vi "FR Measure.vi"(11 "FFmeter settings":T1={"AC Source"={"AC Source type"=enum."Fluke 5XXX calibrator", "VISA"="", "Ref. clock (Hz)"=0.0, "status ref"=refnum}, "TWM pipe"="\\\\.\\pipe\\TWM:server", "Measurement status ref"=refnum, "TWM Status ref"=refnum, "Abort ref"=refnum, "DC meter"={"DC meter type"=enum."H/A/K 3458", "DC meter VISA"="", "NPLC"=10, "status ref"=refnum}, "Measurement properties"={"Measurement frequencies (Hz)"=[1000.0], "Sampling frequency (Hz)"=500000.0, "Signal amplitude (V)"=4.5, "AC-DC settle time (s)"=20.0, "Record length (multiples of period)"=[1000.0, 10000.0, 1000.0], "Measurement template file"=path "", "Row of START keyword"=1, "Row of STOP keyword"=0, "Calculate RMS from samples"=FALSE, "AC-DC warm up time (s)"=300.0, "Measurement template line"=[], "DC meter readings No."=10, "Algorithm"="TWM-WFFT"}, "Skip waiting ref"=refnum, "Octave paths"={"GNU Octave path"=path "C:/Program Files/GNU Octave/Octave-6.2.0/mingw64/bin", "TWM+QWTB path"=path "C:/Users/labina/Desktop/TWM-1.8.7.0-full/octprog", "lvlib path"=path "D:/martin/WAC/WACsw - github/control_software/Filter function meter/external libraries/GOLPI 0.7.3.1 source distribution LV 20.0 32 bit/lv_proc.dll"}, "Template definition"={"Keywords column"=0, "Sig. freq. column"=1, "Rec. len. column"=2, "Meas. points. row min to read"=9, "Meas. points. row max to read"=1509, "Properties column"=4, "Properties row start"=1, "Properties row end"=5, "Keyword START regexp"="", "Keyword STOP regexp"="", "HW data column"=7, "HW data row start"=1, "HW data row end"=3, "TIme and date column start"=3, "Digitizer value column start "=4, "DC mean column start "=6, "DC readings column start"=10}} {"Measurement properties"."Record length (multiples of period)" format="%#_3p"; "Measurement properties"."Sampling frequency (Hz)" format="%#_3p"; "Measurement properties"."Measurement frequencies (Hz)" format="%#_3p"}) -> (0 "error out":errorcluster, 3 "FFmeter settings out":T1={"AC Source"={"AC Source type"=enum."Fluke 5XXX calibrator", "VISA"="", "Ref. clock (Hz)"=0.0, "status ref"=refnum}, "TWM pipe"="\\\\.\\pipe\\TWM:server", "Measurement status ref"=refnum, "TWM Status ref"=refnum, "Abort ref"=refnum, "DC meter"={"DC meter type"=enum."H/A/K 3458", "DC meter VISA"="", "NPLC"=10, "status ref"=refnum}, "Measurement properties"={"Measurement frequencies (Hz)"=[1000.0], "Sampling frequency (Hz)"=500000.0, "Signal amplitude (V)"=4.5, "AC-DC settle time (s)"=20.0, "Record length (multiples of period)"=[1000.0, 10000.0, 1000.0], "Measurement template file"=path "", "Row of START keyword"=1, "Row of STOP keyword"=0, "Calculate RMS from samples"=FALSE, "AC-DC warm up time (s)"=300.0, "Measurement template line"=[], "DC meter readings No."=10, "Algorithm"="TWM-WFFT"}, "Skip waiting ref"=refnum, "Octave paths"={"GNU Octave path"=path "C:/Program Files/GNU Octave/Octave-6.2.0/mingw64/bin", "TWM+QWTB path"=path "C:/Users/labina/Desktop/TWM-1.8.7.0-full/octprog", "lvlib path"=path "D:/martin/WAC/WACsw - github/control_software/Filter function meter/external libraries/GOLPI 0.7.3.1 source distribution LV 20.0 32 bit/lv_proc.dll"}, "Template definition"={"Keywords column"=0, "Sig. freq. column"=1, "Rec. len. column"=2, "Meas. points. row min to read"=9, "Meas. points. row max to read"=1509, "Properties column"=4, "Properties row start"=1, "Properties row end"=5, "Keyword START regexp"="", "Keyword STOP regexp"="", "HW data column"=7, "HW data row start"=1, "HW data row end"=3, "TIme and date column start"=3, "Digitizer value column start "=4, "DC mean column start "=6, "DC readings column start"=10}} {"Measurement properties"."Record length (multiples of period)" format="%#_3p"; "Measurement properties"."Sampling frequency (Hz)" format="%#_3p"; "Measurement properties"."Measurement frequencies (Hz)" format="%#_3p"})   [LabVIEW 2020]
uses:
  FR GUI/Type definitions/FFmeter settings.ctl
  General AC source/Type definitions/AC Source.ctl
  General AC source/Type definitions/AC Source type.ctl
  General DC meter/Type definitions/DC meter.ctl
  General DC meter/Type definitions/DC meter type.ctl
  Type definitions/FR Measuement properties.ctl
  FR Utilities/Type definitions/FR Template definition.ctl
  <vilib>/Utility/error.llb/DialogType.ctl
  external libraries/TWM-1.8.7.0-client/TWM Client Quantity Record.ctl
  <vilib>/Utility/NIReport.llb/NI_report.lvclass
  external libraries/varilib/varilib.lvlib
  external libraries/TWM-1.8.7.0-client/TWM Client.lvlib
panel:
  out "DC readings of AC-AC sequence":dbl[][](array[numeric])
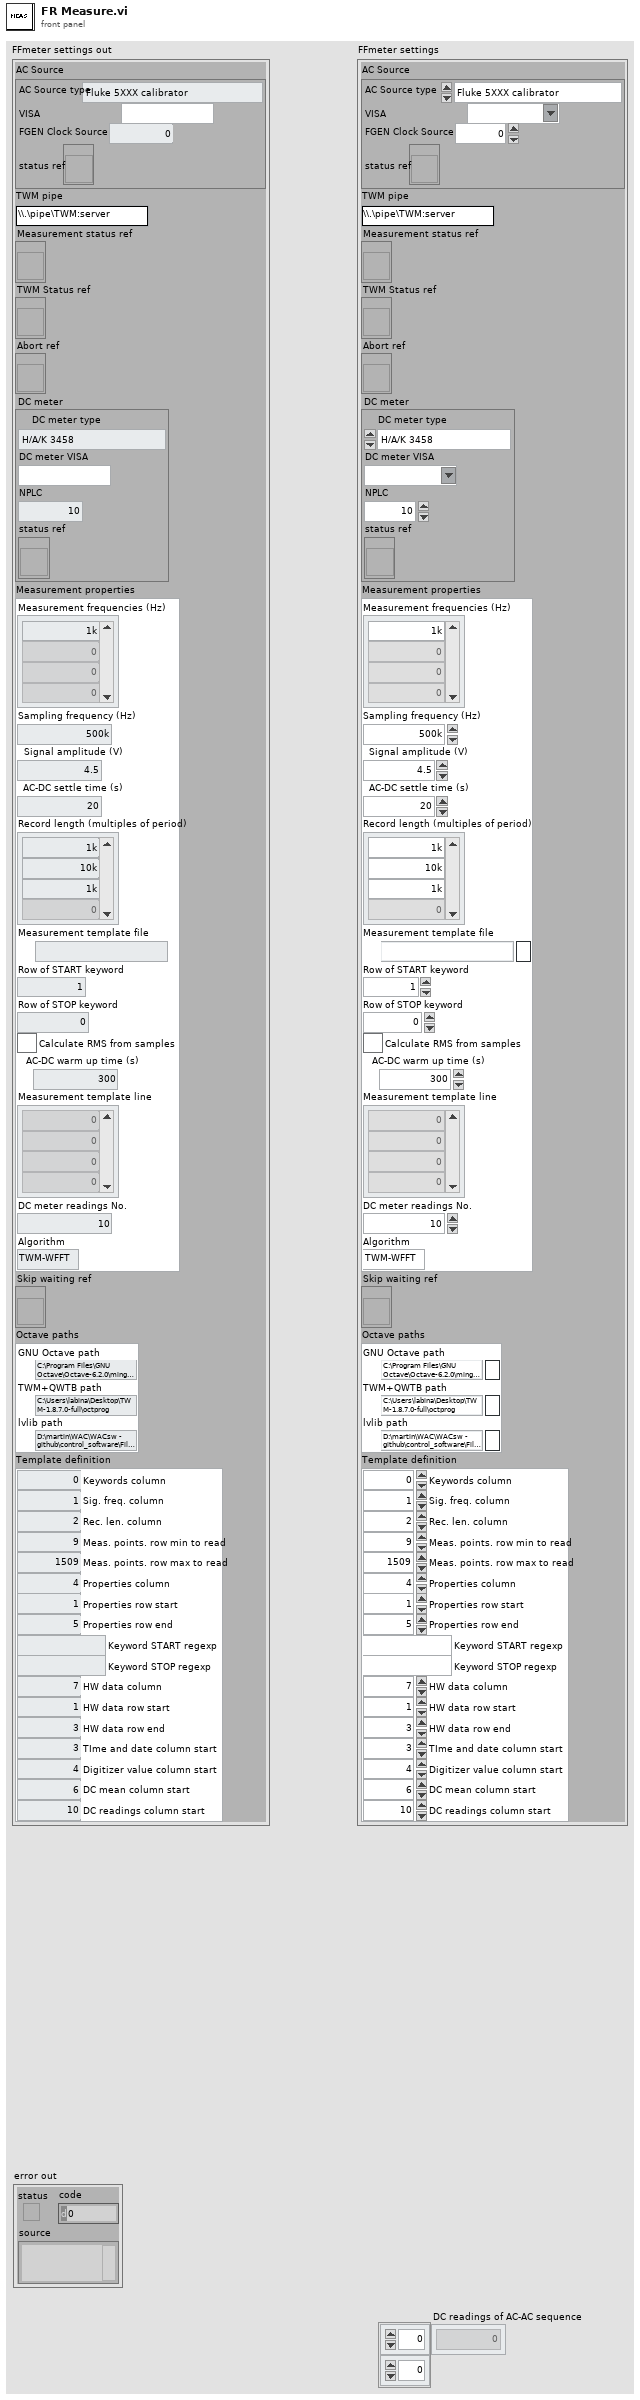
[diagram p1: front panel]
types:
  T1 = typedef "FFmeter settings.ctl" = cluster{"AC Source":T2, "TWM pipe":string, "Measurement status ref":refnum<vi>, "TWM Status ref":refnum<vi>, "Abort ref":refnum<vi>, "DC meter":T4, "Measurement properties":T6, "Skip waiting ref":refnum<vi>, "Octave paths":cluster{"GNU Octave path":path, "TWM+QWTB path":path, "lvlib path":path}, "Template definition":T7}
  T2 = typedef "AC Source.ctl" = cluster{"AC Source type":T3, "VISA":refnum<visa-resource-name>, "Ref. clock (Hz)":dbl, "status ref":refnum<vi>}
  T3 = typedef "AC Source type.ctl" = enum16{"Fluke 5XXX calibrator", "Tektronix AFG3000 series", "dummy"}
  T4 = typedef "DC meter.ctl" = cluster{"DC meter type":T5, "DC meter VISA":refnum<visa-resource-name>, "NPLC":i32, "status ref":refnum<vi>}
  T5 = typedef "DC meter type.ctl" = enum16{"H/A/K 3458", "FLuke 8508A", "dummy"}
  T6 = typedef "FR Measuement properties.ctl" = cluster{"Measurement frequencies (Hz)":dbl[], "Sampling frequency (Hz)":dbl, "Signal amplitude (V)":dbl, "AC-DC settle time (s)":dbl, "Record length (multiples of period)":dbl[], "Measurement template file":path, "Row of START keyword":i32, "Row of STOP keyword":i32, "Calculate RMS from samples":bool, "AC-DC warm up time (s)":dbl, "Measurement template line":i32[], "DC meter readings No.":i32, "Algorithm":string}
  T7 = typedef "FR Template definition.ctl" = cluster{"Keywords column":i32, "Sig. freq. column":i32, "Rec. len. column":i32, "Meas. points. row min to read":i32, "Meas. points. row max to read":i32, "Properties column":i32, "Properties row start":i32, "Properties row end":i32, "Keyword START regexp":string, "Keyword STOP regexp":string, "HW data column":i32, "HW data row start":i32, "HW data row end":i32, "TIme and date column start":i32, "Digitizer value column start ":i32, "DC mean column start ":i32, "DC readings column start":i32}
  T8 = typedef "DialogType.ctl" = u16
  T9 = typedef "TWM Client.lvlib/TWM Client Quantity Record.ctl" = cluster{"val":dbl[], "unc":dbl[], "name":string, "is valid?":bool, "has unc?":bool, "numel":i32, "ua":dbl[], "is phase?":bool, "is amplitude?":bool, "description":string, "phase tag":string, "num format":string, "is string?":bool, "string value":string}
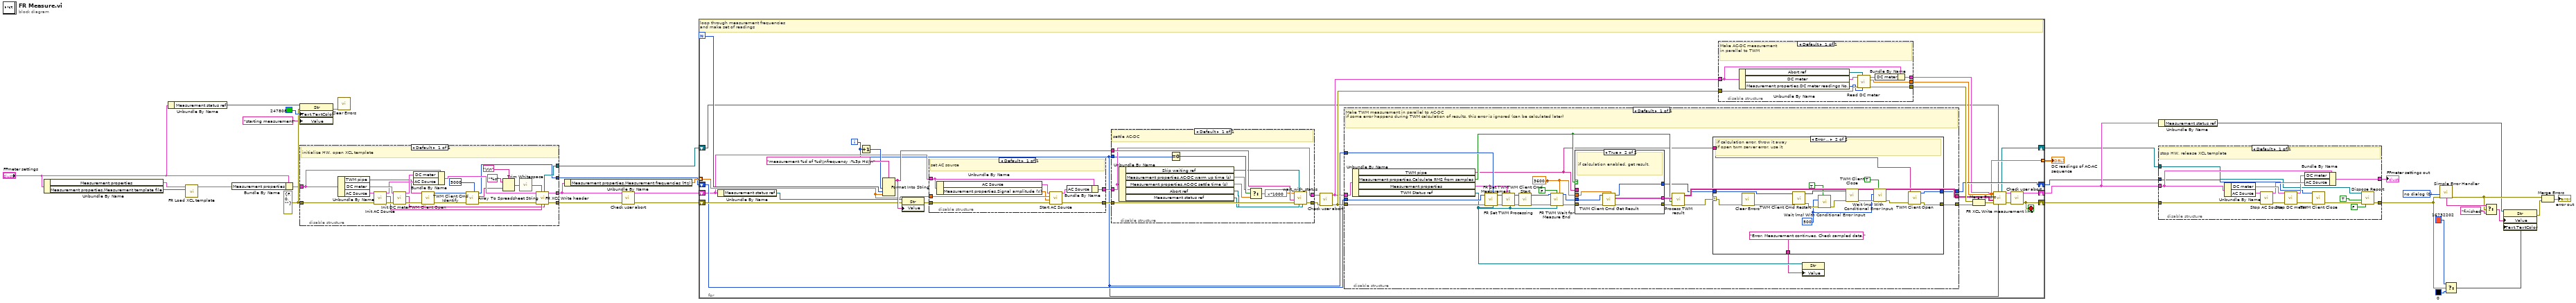
[diagram p0: block diagram]
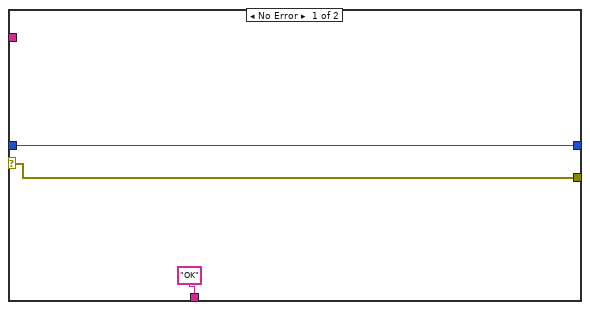
[diagram p2: hidden frame]
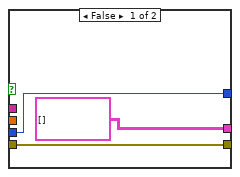
[diagram p3: hidden frame]
diagram:
  w30 = T8 0 items=["no dialog", "OK message", "continue or stop message", "OK message + warnings", "continue/stop + warnings"] ("type of dialog (OK msg:1)")
  w10 = errorcluster {"status"=FALSE, "code"=0, "source"=""} ("error out")
  n1 = Unbundle By Name("FFmeter settings") -> ("Measurement properties"=w8:T6, "Measurement properties.Measurement template file"=w4:path)
  n2 = Unbundle By Name("FFmeter settings") -> ("Measurement status ref"=w22:refnum<vi>)
  n3 = call "FR Load XCL template.vi"("Measurement template file"=w4, "Measurement properties"=w8) -> ("Measurement properties out"=w7:T6)  [unwired: 9 in]
  n4 = Bundle By Name(cluster="FFmeter settings", "Measurement properties"=w7) -> (w5:T1)
  n5 = property class="Str"(reference=w22, error in=w10, "Text.TextColor"=u32 247808 ("Text.Text Colors:Text Color"), "Value"="starting measurement") -> (error out=w21:errorcluster)  [unwired: 1 out]
  n6 = disable-structure shown="Default" {
    disable-tunnel: w5 -> [w57]
    disable-tunnel: [w48] -> w1
    disable-tunnel: w10 -> [w54]
    disable-tunnel: [w51] -> w2
    disable-tunnel: [w39] -> w3
    disable-tunnel: [w49] -> w12
    frame Enabled {
      # "initialize HW, open XCL template"
      n7 = Unbundle By Name(w57) -> ("TWM pipe"=w52:string, "DC meter"=w58:T4, "AC Source"=w59:T2)
      n8 = call "Init AC Source.vi"("error in (no error)"=w54, "AC source"=w59) -> ("error out"=w60:errorcluster, "Init status"=w47:string, "AC source out"=w55:T2)  [unwired: 7 in]
      n9 = call "Init DC meter.vi"("error in (no error)"=w60, "DC meter"=w58) -> ("error out"=w53:errorcluster, "Init status"=w46:string, "DC meter out"=w56:T4)  [unwired: 7 in]
      n10 = Bundle By Name(cluster=w57, "DC meter"=w56, "AC Source"=w55) -> (w50:T1)
      n11 = call "TWM Client Open.vi"("error in"=w53, "pipe name"=w52) -> ("error out"=w41:errorcluster, "handle out"=w42:i32)  [unwired: 8 in]
      n12 = call "TWM Client Cmd Identify.vi"("timeout [ms]"=5000, "error in"=w41, "handle"=w42) -> ("error out"=w40:errorcluster, "channel idns"=w45:string[], "handle out"=w39:i32)  [unwired: 5 in, 1 out]
      n13 = Array To Spreadsheet String(delimiter (Tab)="\r\n", array=w45, 3:"%s" ("format string")) -> (spreadsheet string=w38:string)
      n14 = call <vilib>:"Trim Whitespace.vi"("string"=w38) -> ("trimmed string"=w37:string)  [unwired: 1 in]
      n15 = call "FR XCL Write header.vi"("DC meter idn"=w46, "AC source idn"=w47, "Digitizer idn"=w37, "error in (no error)"=w40, "FFmeter settings"=w50) -> ("error out"=w51:errorcluster, "FFmeter settings out"=w48:T1, "NI_report out"=w49:refnum<class "NI_report.lvclass">)  [unwired: 4 in]
    }
  }
  n16 = call <vilib>:"Clear Errors.vi"("error in (no error)"=w21) -> ()  [unwired: 5 in, 2 out]
  n17 = Unbundle By Name(w1) -> ("Measurement properties.Measurement frequencies (Hz)"=w35:dbl[])
  n18 = call "Check user abort.vi"("error in (no error)"=w2, "FFmeter settings"=w1) -> ("error out"=w20:errorcluster, "FFmeter settings out"=w19:T1)  [unwired: 8 in]
  n19 = for {
    N -> [w87]
    shift-right: [w74] -> w17
    shift-left: w20 -> [w79]
    shift-right: [w73] -> w15
    shift-left: w19 -> [w62]
    tunnel: w35 -> [w80] mode=indexing
    tunnel: [w70] -> w34 mode=indexing
    shift-right: [w66] -> w11
    shift-left: w12 -> [w65]
    shift-right: [w72] -> w13
    shift-left: w3 -> [w63]
    i -> [w61]
    stop <- w74 stop-if-true
    # "loop through measurement frequencies\nand make set of readings"
    n20 = Unbundle By Name(w62) -> ("Measurement status ref"=w84:refnum<vi>)
    n21 = Increment(x=w61) -> (x+1=w88:i32)
    n22 = Format Into String(format string="measurement %d of %d\\nfrequency :%3p Hz\\n", w88, w87, w80) -> (resulting string=w89:string)  [unwired: 2 in, 1 out]
    n23 = property class="Str"(reference=w84, error in=w79, "Value"=w89) -> (error out=w83:errorcluster)  [unwired: 1 out]
    n24 = disable-structure shown="Default" {
      disable-tunnel: w62 -> [w110]
      disable-tunnel: w83 -> [w109]
      disable-tunnel: [w108] -> w82
      disable-tunnel: [w111] -> w81
      disable-tunnel: w80 -> [w105]
      frame Enabled {
        # "set AC source"
        n25 = Unbundle By Name(w110) -> ("AC Source"=w106:T2, "Measurement properties.Signal amplitude (V)"=w104:dbl)
        n26 = call "Start AC Source.vi"("error in (no error)"=w109, "Signal amplitude (V)"=w104, "Signal frequency  (Hz)"=w105, "AC source"=w106) -> ("error out"=w108:errorcluster, "AC source out"=w107:T2)  [unwired: 5 in, 1 out]
        n27 = Bundle By Name(cluster=w110, "AC Source"=w107) -> (w111:T1)
      }
    }
    n28 = disable-structure shown="Default" {
      disable-tunnel: w89 -> [w103]
      disable-tunnel: [w97] -> w78
      disable-tunnel: [w101] -> w75
      disable-tunnel: w82 -> [w102]
      disable-tunnel: w81 -> [w101]
      disable-tunnel: w61 -> [w96]
      frame Enabled {
        # "settle AC-DC"
        n29 = Unbundle By Name(w101) -> ("Skip waiting ref"=w91:refnum<vi>, "Measurement properties.AC-DC warm up time (s)"=w94:dbl, "Measurement properties.AC-DC settle time (s)"=w93:dbl, "Abort ref"=w99:refnum<vi>, "Measurement status ref"=w98:refnum<vi>)
        n30 = Equal To 0?(x=w96) -> (x = 0?=w95:bool)
        n31 = Select(t=w94, s=w95, f=w93) -> (s? t:f=w92:dbl)
        n32 = expression code="x*1000"(w92) -> (w100:dbl)
        n33 = call "wait_with_status.vi"("stat ref"=w98, "stop ref"=w99, "second stop ref"=w91, "error in"=w102, "comment"=w103, "ms to wait"=w100) -> ("error out"=w97:errorcluster)  [unwired: 4 in, 1 out]
      }
    }
    n34 = call "Check user abort.vi"("error in (no error)"=w78, "FFmeter settings"=w75) -> ("error out"=w77:errorcluster, "FFmeter settings out"=w76:T1)  [unwired: 8 in]
    n35 = disable-structure shown="Default" {
      disable-tunnel: [w131] -> w85
      disable-tunnel: w77 -> [w142]
      disable-tunnel: w76 -> [w146]
      disable-tunnel: w63 -> [w141]
      disable-tunnel: [w127] -> w72
      disable-tunnel: w61 -> [w145]
      disable-tunnel: [w135] -> w64
      frame Enabled {
        w126 = 3600.0 ("timeout [s] (10s)")
        # "Make TWM measurement in parallel to AC-DC\nif some error happens during TWM calculation of results, this error is ignored (can be calculated later)"
        n36 = Unbundle By Name(w146) -> ("TWM pipe"=w121:string, "Measurement properties.Calculate RMS from samples"=w133:bool, "Measurement properties"=w136:T6, "TWM Status ref"=w123:refnum<vi>)
        n37 = call "FR Set TWM Measurement.vi"("status ref (none)"=w123, "Loop iteration"=w145, "Measurement properties"=w136, "error in"=w142, "handle"=w141) -> ("error out"=w140:errorcluster, "handle out"=w137:i32)  [unwired: 5 in]
        n38 = call "FR Set TWM Processing.vi"("status ref (none)"=w123, "Measurement properties"=w136, "error in"=w140, "handle"=w137) -> ("error out"=w139:errorcluster, "handle out"=w138:i32)  [unwired: 6 in]
        n39 = call "TWM Client Cmd Start.vi"("error in"=w139, "handle"=w138) -> ("error out"=w144:errorcluster, "handle out"=w143:i32)  [unwired: 8 in]
        n40 = call "FR TWM Wait for Measure End.vi"("handle"=w143, "Obtain results? (False)"=FALSE, "timeout [s] (10s)"=w126, "error in"=w144, "status ref (none)"=w123) -> ("handle out"=w129:i32, "error out"=w130:errorcluster)  [unwired: 6 in, 3 out]
        n41 = case shown="True" w133 {
          tunnel: [T9[][] [] ("result data") w173] -> w134
          tunnel: w129 -> [w166 w172]
          tunnel: w121 -> [_ _]
          tunnel: w130 -> [w165 w171]
          tunnel: [w166 w170] -> w128
          tunnel: w126 -> [_ w169]
          tunnel: [w165 w168] -> w125
          frame False {
          }
          frame True {
            # "if calculation enabled, get result."
            n42 = call "TWM Client Cmd Get Result.vi"("timeout [s] (10s)"=w169, "error in"=w171, "handle"=w172) -> ("error out"=w168:errorcluster, "result data"=w173:T9[][], "handle out"=w170:i32)  [unwired: 5 in, 1 out]
          }
        }
        n43 = call "Process TWM result.vi"("error from TWM get result"=w125, "Calculate RMS from samples"=w133, "TWM result"=w134) -> ("error out"=w124:errorcluster, "TWM result as string for XCL"=w135:string[][])  [unwired: 7 in]
        n44 = case shown="Error .." w124 {
          selector: w124 -> [w149 w164]
          tunnel: [w149 w160] -> w131
          tunnel: w128 -> [w148 w163]
          tunnel: [w148 w159] -> w127
          tunnel: ["OK" ("Value") "Error. Measurement continues. Check sampled data." ("Value")] -> w122
          tunnel: w121 -> [_ w150]
          frame No Error {
          }
          frame Error {
            w152 = u32 500 ("milliseconds to wait")
            # "if calculation error, throw it away\nif open twm server error, use it"
            n45 = call <vilib>:"Clear Errors.vi"("error in (no error)"=w164) -> ("error out"=w162:errorcluster)  [unwired: 5 in, 1 out]
            n46 = call "TWM Client Cmd Restart.vi"("error in"=w162, "handle"=w163) -> ("error out"=w158:errorcluster, "handle out"=w161:i32)  [unwired: 8 in]
            n47 = call "Wait (ms) With Conditional Error Input.vi"("wait if error (F)"=TRUE, "error in (no error)"=w158, "milliseconds to wait"=w152) -> ("error out"=w157:errorcluster)  [unwired: 7 in, 1 out]
            n48 = call "TWM Client Close.vi"("error in"=w157, "handle in"=w161) -> ("error out"=w156:errorcluster)  [unwired: 9 in]
            n49 = call "Wait (ms) With Conditional Error Input.vi"("wait if error (F)"=TRUE, "error in (no error)"=w156, "milliseconds to wait"=w152) -> ("error out"=w155:errorcluster)  [unwired: 7 in, 1 out]
            n50 = call "TWM Client Open.vi"("error in"=w155, "pipe name"=w150) -> ("error out"=w160:errorcluster, "handle out"=w159:i32)  [unwired: 8 in]
          }
        }
        n51 = property class="Str"(reference=w123, "Value"=w122) -> ()  [unwired: 1 in, 2 out]
      }
    }
    n52 = disable-structure shown="Default" {
      disable-tunnel: [w120] -> w70
      disable-tunnel: [w119] -> w86
      disable-tunnel: w77 -> [w118]
      disable-tunnel: w76 -> [w115]
      disable-tunnel: [w114] -> w71
      frame Enabled {
        # "Make AC-DC measurement\nin parallel to TWM"
        n53 = Unbundle By Name(w115) -> ("Abort ref"=w113:refnum<vi>, "DC meter"=w117:T4, "Measurement properties.DC meter readings No."=w112:i32)
        n54 = call "Read DC meter.vi"("No of readings"=w112, "abort reference"=w113, "error in (no error)"=w118, "DC meter"=w117) -> ("error out"=w119:errorcluster, "DC readings"=w120:dbl[], "DC meter out"=w116:T4)  [unwired: 5 in]
        n55 = Bundle By Name(cluster=w115, "DC meter"=w116) -> (w114:T1)
      }
    }
    n56 = Merge Errors(w86, w85) -> (w69:errorcluster)
    n57 = call "FR XCL Write measurement line.vi"("Iteration index"=w61, "report in"=w65, "error in (no error)"=w69, "TWM result as string for XCL"=w64, "DC readings"=w70, "FFmeter settings in"=w71) -> ("error out"=w68:errorcluster, "FFmeter settings out"=w67:T1, "report out"=w66:refnum<class "NI_report.lvclass">)  [unwired: 3 in]
    n58 = call "Check user abort.vi"("error in (no error)"=w68, "FFmeter settings"=w67) -> ("error out"=w74:errorcluster, "FFmeter settings out"=w73:T1)  [unwired: 8 in]
  }
  "DC readings of AC-AC sequence" <- w34
  n59 = Unbundle By Name(w15) -> ("Measurement status ref"=w18:refnum<vi>)
  n60 = disable-structure shown="Default" {
    disable-tunnel: w15 -> [w188]
    disable-tunnel: [w187] -> w14
    disable-tunnel: [w177] -> w16
    disable-tunnel: w17 -> [w181]
    disable-tunnel: w13 -> [w179]
    disable-tunnel: w11 -> [w176]
    frame Enabled {
      # "stop HW, release XCL template"
      n61 = Unbundle By Name(w188) -> ("DC meter"=w184:T4, "AC Source"=w185:T2)
      n62 = call "Stop AC Source.vi"("error in (no error)"=w181, "AC source"=w185) -> ("error out"=w186:errorcluster, "AC source out"=w183:T2)  [unwired: 8 in]
      n63 = call "Stop DC meter.vi"("error in (no error)"=w186, "DC meter"=w184) -> ("error out"=w180:errorcluster, "DC meter out"=w182:T4)  [unwired: 8 in]
      n64 = Bundle By Name(cluster=w188, "DC meter"=w182, "AC Source"=w183) -> (w187:T1)
      n65 = call "TWM Client Close.vi"("error in"=w180, "handle in"=w179) -> ("error out"=w178:errorcluster)  [unwired: 9 in]
      n66 = call-dynamic "Dispose Report.vi"("report in"=w176, "save changes? (F)"=TRUE, "error in (no error)"=w178, "close report? (T)"=FALSE) -> ("error out"=w177:errorcluster)  [unwired: 11 in]
    }
  }
  "FFmeter settings out" <- w14
  n67 = call <vilib>:"Simple Error Handler.vi"("type of dialog (OK msg:1)"=w30, "error in (no error)"=w16) -> ("error out"=w25:errorcluster, "message"=w33:string)  [unwired: 3 in, 3 out]
  n68 = Select(t=u32 16732202 ("Text.Text Colors:Text Color"), s=w16, f=u32 0 ("Text.Text Colors:Text Color")) -> (s? t:f=w27:u32)
  n69 = Select(t=w33, s=w25, f="finished") -> (s? t:f=w31:string)
  n70 = property class="Str"(reference=w18, "Value"=w31, "Text.TextColor"=w27) -> (error out=w26:errorcluster)  [unwired: 1 in, 1 out]
  n71 = Merge Errors(w25, w26) -> (→"error out":errorcluster)
